vi "FPGAvi.vi"() -> ()   [LabVIEW 2014]
uses:
  <vilib>/Platform/TimedLoop/XDataNode/wakeup.ctl
  <vilib>/Platform/TimedLoop/XDataNode/XDNodeRunTimeDep.lvlib
  <vilib>/Platform/TimedLoop/XDataNode/nitl_modes.ctl
  <vilib>/Platform/TimedLoop/XDataNode/timing_clust.ctl
  <vilib>/Platform/TimedLoop/XDataNode/XDataNode.xnode
  <vilib>/eio/EIONode/EIONode.xnode
  <vilib>/rvi/eio/common/nirviEmuTemplateMethod_errors.vi
  <vilib>/rvi/DataTransferAndStorage/Container/XNode/niFpgaContainer.xnode
  <vilib>/rvi/FIFO/Fifo_Resource/nirvififoEmulationWrite.vi
  <vilib>/rvi/FIFO/Fifo_Resource/nirvififoEmulationRead.vi
  <vilib>/rvi/interface/RandomDataEmulation/nirviRandomDataFpgaReadWriteTemplate.vi
panel:
  out "DMA Overflow":bool
  in  "ADC A Requested":bool
  in  "ADC B Requested":bool
  in  "ADC C Requested":bool
  in  "ADC D Requested":bool
  in  "Acquire":bool
  out "Acquisition State":T1(ring)
  out "FIFO State":T2(ring)
  out "Init Done":bool
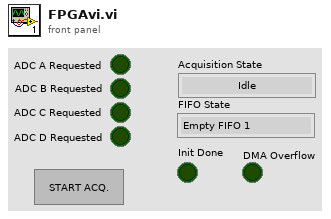
[diagram p1: front panel]
types:
  T1 = enum16{"Idle", "Determine Channel Selection", "Acquire", "Transfer"}
  T2 = enum16{"Empty FIFO 1", "Empty FIFO 2", "Empty FIFO 3", "Empty FIFO 4", "Empty FIFO 5", "Empty FIFO 6", "Empty FIFO 7", "Empty FIFO 8", "FIFO Read Complete"}
  T3 = typedef "XDNodeRunTimeDep.lvlib/timing_clust.ctl" = cluster{"Expected End [f-1]":u64, "Actual End [f-1]":u64, "Finished Late? [f-1]":bool, "Expected End [i-1]":u64, "Actual End [i-1]":u64, "Finished Late? [i-1]":bool, "Expected Start [i]":u64, "Actual Start [i]":u64, "Expected Start [f]":u64, "Actual Start [f]":u64, "Source Name":string, "Structure Name":string, "Period":i64, "Deadline":i64, "Offset":i64, "Start":i64, "Priority":i32, "Timeout":i32, "Mode":T4, "Wakeup Reason":T5, "Error":errorcluster, "Source Type":string, "Secondary Source Type":string, "Global End Time":u64, "Global Start Time":u64, "Frame Duration":u64, "Iteration Duration":u64, "Assigned CPU":i32, "I/O Scan Engine Mode":u32}
  T4 = typedef "XDNodeRunTimeDep.lvlib/nitl_modes.ctl" = enum32{"No Change", "Process missed periods, maintain original phase", "Discard missed periods, maintain original phase", "Process missed periods, ignore original phase", "Discard missed periods, ignore original phase"}
  T5 = typedef "XDNodeRunTimeDep.lvlib/wakeup.ctl" = enum32{"Normal", "Aborted", "Asynchronous wakeup", "Timing source error", "Timed loop error", "Timeout"}
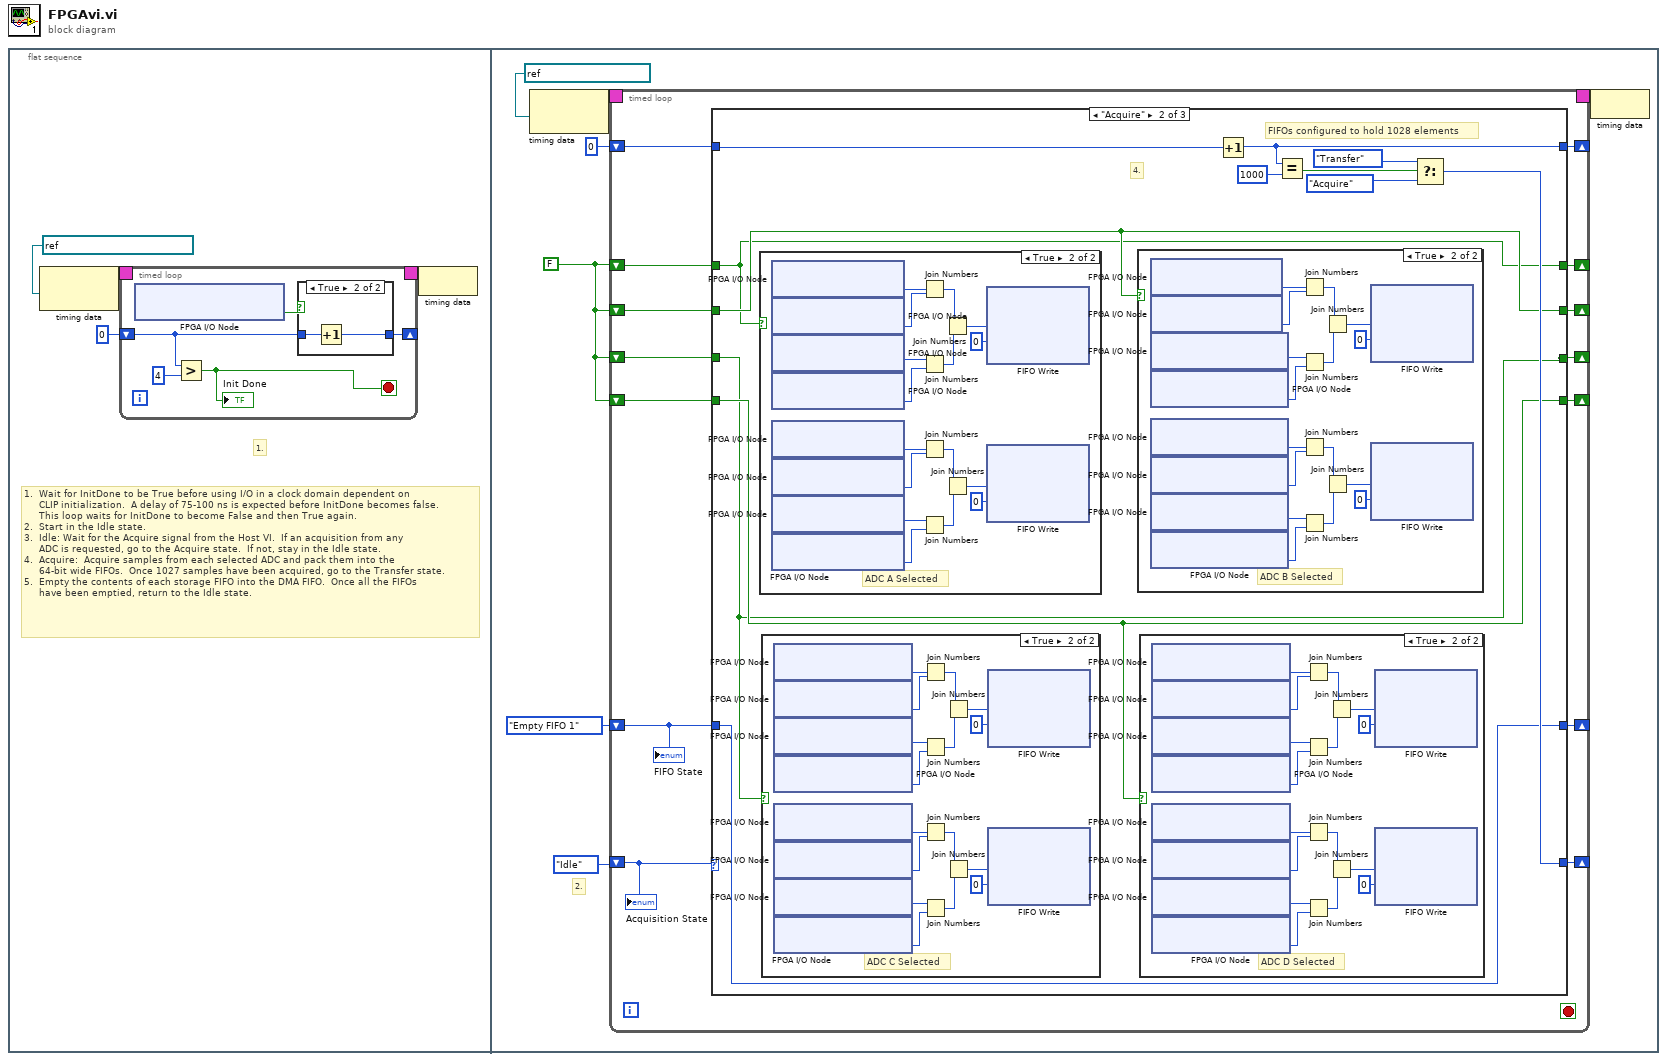
[diagram p0: block diagram]
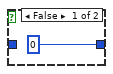
[diagram p2: hidden frame]
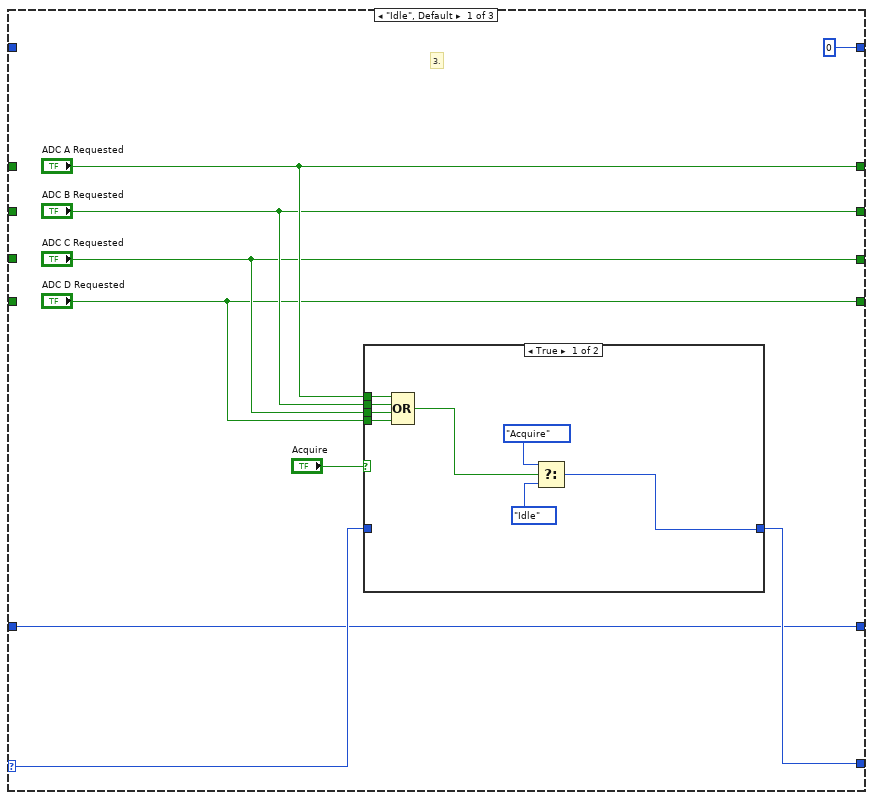
[diagram p3: hidden frame]
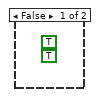
[diagram p5: hidden frame]
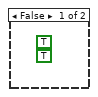
[diagram p6: hidden frame]
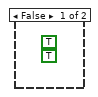
[diagram p7: hidden frame]
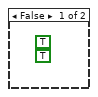
[diagram p8: hidden frame]
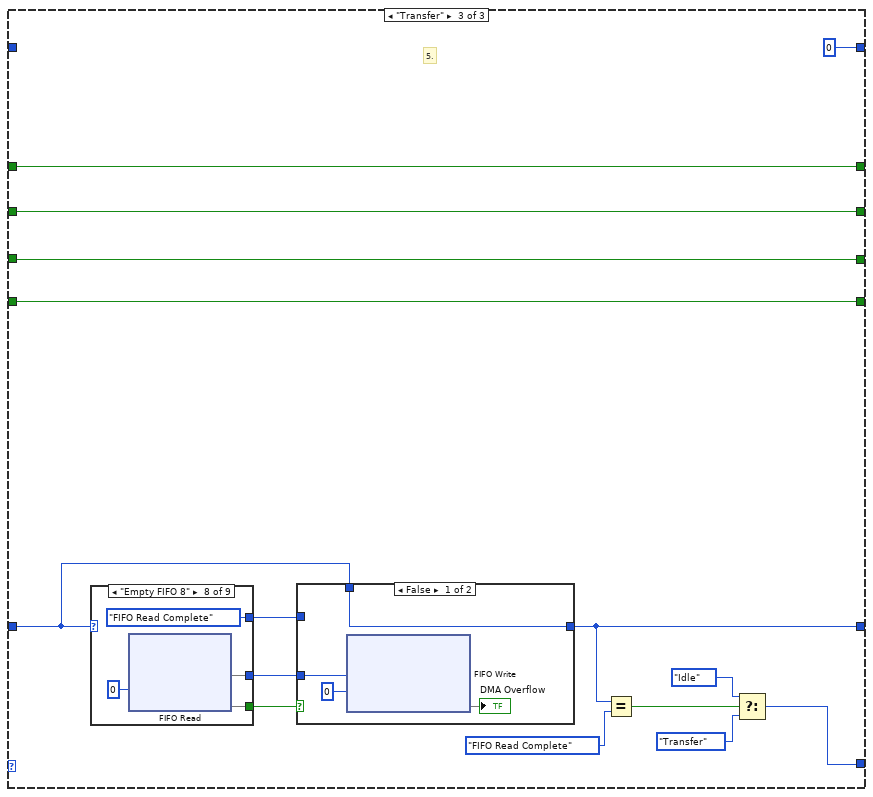
[diagram p9: hidden frame]
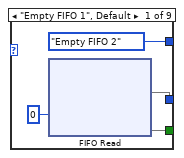
[diagram p11: hidden frame]
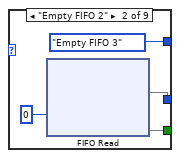
[diagram p12: hidden frame]
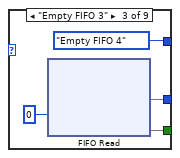
[diagram p13: hidden frame]
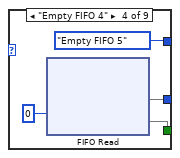
[diagram p14: hidden frame]
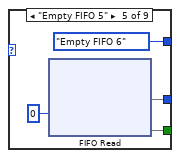
[diagram p15: hidden frame]
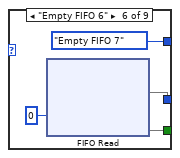
[diagram p16: hidden frame]
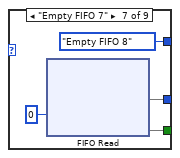
[diagram p17: hidden frame]
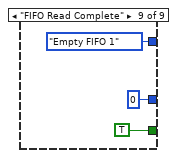
[diagram p18: hidden frame]
diagram:
  n1 = flat-sequence {
    frame #0 {
      # "1.  Wait for InitDone to be True before using I/O in a clock domain dependent on \n     CLIP initialization.  A delay of 75-100 ns is expected before InitDone becomes false.  \n     This loop waits for InitDone to become False and then True again.\n2.  Start in the Idle state. \n3.  Idle: Wait for the Acquire signal from the Host VI.  If an acquisition from any \n     ADC is requested, go to the Acquire state.  If not, stay in the Idle state.\n4.  Acquire:  Acquire samples from each selected ADC and pack them into the  \n     64-bit wide FIFOs.  Once 1027 samples have been acquired, go to the Transfer state.\n5.  Empty the contents of each storage FIFO into the DMA FIFO.  Once all the FIFOs \n     have been emptied, return to the Idle state."
      # "1."
      n2 = node-c288(refnum<k21> "40 MHz Onboard Clock" ("Source Name")) -> (w4:T3)
      n3 = timed-loop {
        shift-right: [w8] -> _
        shift-left: u16 0 -> [w7]
        timing: w4 -> [_]
        timing-out: [_] -> w3
        stop <- w5 stop-if-true
        n4 = xnode "FPGA I/O Node"() -> ("IO Module\\InitDone"=w9:bool)  [unwired: 1 in, 1 out]
        n5 = Greater?(x=w7, y=u16 4) -> (0:w5:bool)
        "Init Done" <- w5
        n6 = case shown="True" w9 {
          tunnel: [u16 0 w12] -> w8
          tunnel: w7 -> [_ w11]
          frame False {
          }
          frame True {
            n7 = Increment(x=w11) -> (x+1=w12:u16)
          }
        }
      }
      n8 = node-c288(w3) -> ()
    }
    frame #1 {
      w22 = FALSE
      # "2."
      n9 = node-c288(refnum<k21> "IO Module Clock 0" ("Source Name")) -> (w25:T3)
      n10 = timed-loop {
        timing: w25 -> [_]
        timing-out: [_] -> w24
        shift-right: [w31] -> _
        shift-left: T1."Idle" ("Acquisition State 2") -> [w28]
        shift-right: [w39] -> _
        shift-left: w22 -> [w35]
        shift-right: [w38] -> _
        shift-left: w22 -> [w34]
        shift-right: [w37] -> _
        shift-left: w22 -> [w33]
        shift-right: [w36] -> _
        shift-left: w22 -> [w32]
        shift-right: [w29] -> _
        shift-left: i16 0 -> [w30]
        shift-right: [w26] -> _
        shift-left: T2."Empty FIFO 1" -> [w27]
        stop <- _ stop-if-true
        n11 = case shown="\"Acquire\"" w28 {
          selector: w28 -> [w43 _ _]
          tunnel: [w48 w67 w137] -> w31
          tunnel: ["ADC A Requested" w59 w148] -> w39
          tunnel: ["ADC B Requested" w60 w147] -> w38
          tunnel: ["ADC C Requested" w61 w146] -> w37
          tunnel: ["ADC D Requested" w62 w145] -> w36
          tunnel: w35 -> [_ w59 w148]
          tunnel: w34 -> [_ w60 w147]
          tunnel: w33 -> [_ w61 w146]
          tunnel: w32 -> [_ w62 w145]
          tunnel: w30 -> [_ w66 _]
          tunnel: [i16 0 w63 i16 0] -> w29
          tunnel: w27 -> [w41 w58 w141]
          tunnel: [w41 w58 w138] -> w26
          frame "Idle", Default {
            # "3."
            n12 = case shown="True" "Acquire" {
              tunnel: "ADC D Requested" -> [w54 _]
              tunnel: "ADC C Requested" -> [w53 _]
              tunnel: "ADC B Requested" -> [w52 _]
              tunnel: "ADC A Requested" -> [w51 _]
              tunnel: [w50 w57] -> w48
              tunnel: w43 -> [_ w57]
              frame True {
                n13 = Compound Arithmetic op=OR(w51, w52, w53, w54) -> (w49:bool)
                n14 = Select(t=T1."Acquire" ("Acquisition State 2"), s=w49, f=T1."Idle" ("Acquisition State 2")) -> (s? t:f=w50:T1)
              }
              frame False {
              }
            }
          }
          frame "Acquire" {
            # "4."
            # "FIFOs configured to hold 1028 elements"
            n15 = case shown="True" w59 {
              frame False {
                (unwired) TRUE ("Timed Out?")
                (unwired) TRUE ("Timed Out?")
              }
              frame True {
                # "ADC A Selected"
                n16 = xnode "FPGA I/O Node"() -> ("IO Module\\AI A0"=w118:i16)  [unwired: 1 in, 1 out]
                n17 = xnode "FPGA I/O Node"() -> ("IO Module\\AI A1"=w119:i16)  [unwired: 1 in, 1 out]
                n18 = xnode "FPGA I/O Node"() -> ("IO Module\\AI A2"=w120:i16)  [unwired: 1 in, 1 out]
                n19 = xnode "FPGA I/O Node"() -> ("IO Module\\AI A3"=w121:i16)  [unwired: 1 in, 1 out]
                n20 = xnode "FPGA I/O Node"() -> ("IO Module\\AI A4"=w122:i16)  [unwired: 1 in, 1 out]
                n21 = xnode "FPGA I/O Node"() -> ("IO Module\\AI A5"=w123:i16)  [unwired: 1 in, 1 out]
                n22 = xnode "FPGA I/O Node"() -> ("IO Module\\AI A6"=w124:i16)  [unwired: 1 in, 1 out]
                n23 = xnode "FPGA I/O Node"() -> ("IO Module\\AI A7"=w125:i16)  [unwired: 1 in, 1 out]
                n24 = Join Numbers(hi=w118, lo=w119) -> ((hi.lo)=w129:u32)
                n25 = Join Numbers(hi=w120, lo=w121) -> ((hi.lo)=w128:u32)
                n26 = Join Numbers(hi=w122, lo=w123) -> ((hi.lo)=w132:u32)
                n27 = Join Numbers(hi=w124, lo=w125) -> ((hi.lo)=w133:u32)
                n28 = Join Numbers(hi=w129, lo=w128) -> ((hi.lo)=w127:u64)
                n29 = Join Numbers(hi=w132, lo=w133) -> ((hi.lo)=w131:u64)
                n30 = xnode ("FIFO Write")("Element"=w127, "Timeout"=0) -> ()  [unwired: 1 in, 2 out]
                n31 = xnode ("FIFO Write")("Element"=w131, "Timeout"=0) -> ()  [unwired: 1 in, 2 out]
              }
            }
            n32 = case shown="True" w61 {
              frame False {
                (unwired) TRUE ("Timed Out?")
                (unwired) TRUE ("Timed Out?")
              }
              frame True {
                # "ADC C Selected"
                n33 = xnode "FPGA I/O Node"() -> ("IO Module\\AI C16"=w86:i16)  [unwired: 1 in, 1 out]
                n34 = xnode "FPGA I/O Node"() -> ("IO Module\\AI C17"=w87:i16)  [unwired: 1 in, 1 out]
                n35 = xnode "FPGA I/O Node"() -> ("IO Module\\AI C18"=w88:i16)  [unwired: 1 in, 1 out]
                n36 = xnode "FPGA I/O Node"() -> ("IO Module\\AI C19"=w89:i16)  [unwired: 1 in, 1 out]
                n37 = xnode "FPGA I/O Node"() -> ("IO Module\\AI C20"=w90:i16)  [unwired: 1 in, 1 out]
                n38 = xnode "FPGA I/O Node"() -> ("IO Module\\AI C21"=w91:i16)  [unwired: 1 in, 1 out]
                n39 = xnode "FPGA I/O Node"() -> ("IO Module\\AI C22"=w92:i16)  [unwired: 1 in, 1 out]
                n40 = xnode "FPGA I/O Node"() -> ("IO Module\\AI C23"=w93:i16)  [unwired: 1 in, 1 out]
                n41 = Join Numbers(hi=w86, lo=w87) -> ((hi.lo)=w97:u32)
                n42 = Join Numbers(hi=w88, lo=w89) -> ((hi.lo)=w96:u32)
                n43 = Join Numbers(hi=w90, lo=w91) -> ((hi.lo)=w100:u32)
                n44 = Join Numbers(hi=w92, lo=w93) -> ((hi.lo)=w101:u32)
                n45 = Join Numbers(hi=w97, lo=w96) -> ((hi.lo)=w95:u64)
                n46 = Join Numbers(hi=w100, lo=w101) -> ((hi.lo)=w99:u64)
                n47 = xnode ("FIFO Write")("Element"=w95, "Timeout"=0) -> ()  [unwired: 1 in, 2 out]
                n48 = xnode ("FIFO Write")("Element"=w99, "Timeout"=0) -> ()  [unwired: 1 in, 2 out]
              }
            }
            n49 = case shown="True" w60 {
              frame False {
                (unwired) TRUE ("Timed Out?")
                (unwired) TRUE ("Timed Out?")
              }
              frame True {
                # "ADC B Selected"
                n50 = xnode "FPGA I/O Node"() -> ("IO Module\\AI B8"=w102:i16)  [unwired: 1 in, 1 out]
                n51 = xnode "FPGA I/O Node"() -> ("IO Module\\AI B9"=w103:i16)  [unwired: 1 in, 1 out]
                n52 = xnode "FPGA I/O Node"() -> ("IO Module\\AI B10"=w104:i16)  [unwired: 1 in, 1 out]
                n53 = xnode "FPGA I/O Node"() -> ("IO Module\\AI B11"=w105:i16)  [unwired: 1 in, 1 out]
                n54 = xnode "FPGA I/O Node"() -> ("IO Module\\AI B12"=w106:i16)  [unwired: 1 in, 1 out]
                n55 = xnode "FPGA I/O Node"() -> ("IO Module\\AI B13"=w107:i16)  [unwired: 1 in, 1 out]
                n56 = xnode "FPGA I/O Node"() -> ("IO Module\\AI B14"=w108:i16)  [unwired: 1 in, 1 out]
                n57 = xnode "FPGA I/O Node"() -> ("IO Module\\AI B15"=w109:i16)  [unwired: 1 in, 1 out]
                n58 = Join Numbers(hi=w102, lo=w103) -> ((hi.lo)=w113:u32)
                n59 = Join Numbers(hi=w104, lo=w105) -> ((hi.lo)=w112:u32)
                n60 = Join Numbers(hi=w106, lo=w107) -> ((hi.lo)=w116:u32)
                n61 = Join Numbers(hi=w108, lo=w109) -> ((hi.lo)=w117:u32)
                n62 = Join Numbers(hi=w113, lo=w112) -> ((hi.lo)=w111:u64)
                n63 = Join Numbers(hi=w116, lo=w117) -> ((hi.lo)=w115:u64)
                n64 = xnode ("FIFO Write")("Element"=w111, "Timeout"=0) -> ()  [unwired: 1 in, 2 out]
                n65 = xnode ("FIFO Write")("Element"=w115, "Timeout"=0) -> ()  [unwired: 1 in, 2 out]
              }
            }
            n66 = case shown="True" w62 {
              frame False {
                (unwired) TRUE ("Timed Out?")
                (unwired) TRUE ("Timed Out?")
              }
              frame True {
                # "ADC D Selected"
                n67 = xnode "FPGA I/O Node"() -> ("IO Module\\AI D24"=w70:i16)  [unwired: 1 in, 1 out]
                n68 = xnode "FPGA I/O Node"() -> ("IO Module\\AI D25"=w71:i16)  [unwired: 1 in, 1 out]
                n69 = xnode "FPGA I/O Node"() -> ("IO Module\\AI D26"=w72:i16)  [unwired: 1 in, 1 out]
                n70 = xnode "FPGA I/O Node"() -> ("IO Module\\AI D27"=w73:i16)  [unwired: 1 in, 1 out]
                n71 = xnode "FPGA I/O Node"() -> ("IO Module\\AI D28"=w74:i16)  [unwired: 1 in, 1 out]
                n72 = xnode "FPGA I/O Node"() -> ("IO Module\\AI D29"=w75:i16)  [unwired: 1 in, 1 out]
                n73 = xnode "FPGA I/O Node"() -> ("IO Module\\AI D30"=w76:i16)  [unwired: 1 in, 1 out]
                n74 = xnode "FPGA I/O Node"() -> ("IO Module\\AI D31"=w77:i16)  [unwired: 1 in, 1 out]
                n75 = Join Numbers(hi=w70, lo=w71) -> ((hi.lo)=w81:u32)
                n76 = Join Numbers(hi=w72, lo=w73) -> ((hi.lo)=w80:u32)
                n77 = Join Numbers(hi=w74, lo=w75) -> ((hi.lo)=w84:u32)
                n78 = Join Numbers(hi=w76, lo=w77) -> ((hi.lo)=w85:u32)
                n79 = Join Numbers(hi=w81, lo=w80) -> ((hi.lo)=w79:u64)
                n80 = Join Numbers(hi=w84, lo=w85) -> ((hi.lo)=w83:u64)
                n81 = xnode ("FIFO Write")("Element"=w79, "Timeout"=0) -> ()  [unwired: 1 in, 2 out]
                n82 = xnode ("FIFO Write")("Element"=w83, "Timeout"=0) -> ()  [unwired: 1 in, 2 out]
              }
            }
            n83 = Increment(x=w66) -> (x+1=w63:i16)
            n84 = Equal?(x=w63, y=i16 1000) -> (x = y?=w64:bool)
            n85 = Select(t=T1."Transfer" ("Acquisition State 2"), s=w64, f=T1."Acquire" ("Acquisition State 2")) -> (s? t:f=w67:T1)
          }
          frame "Transfer" {
            # "5."
            n86 = case shown="\"Empty FIFO 8\"" w141 {
              tunnel: [w156 w160 w163 w166 w171 w175 w180 w182 u64 0 ("Element")] -> w142
              tunnel: [w155 w159 w162 w167 w170 w174 w178 w183 TRUE ("Timed Out?")] -> w143
              tunnel: [T2."Empty FIFO 2" T2."Empty FIFO 3" T2."Empty FIFO 4" T2."Empty FIFO 5" T2."Empty FIFO 6" T2."Empty FIFO 7" T2."Empty FIFO 8" T2."FIFO Read Complete" T2."Empty FIFO 1"] -> w140
              frame "Empty FIFO 1", Default {
                n87 = xnode ("FIFO Read")("Timeout"=0) -> ("Element"=w156, "Timed Out?"=w155)  [unwired: 1 in, 1 out]
              }
              frame "Empty FIFO 2" {
                n88 = xnode ("FIFO Read")("Timeout"=0) -> ("Element"=w160, "Timed Out?"=w159)  [unwired: 1 in, 1 out]
              }
              frame "Empty FIFO 3" {
                n89 = xnode ("FIFO Read")("Timeout"=0) -> ("Element"=w163, "Timed Out?"=w162)  [unwired: 1 in, 1 out]
              }
              frame "Empty FIFO 4" {
                n90 = xnode ("FIFO Read")("Timeout"=0) -> ("Element"=w166, "Timed Out?"=w167)  [unwired: 1 in, 1 out]
              }
              frame "Empty FIFO 5" {
                n91 = xnode ("FIFO Read")("Timeout"=0) -> ("Element"=w171, "Timed Out?"=w170)  [unwired: 1 in, 1 out]
              }
              frame "Empty FIFO 6" {
                n92 = xnode ("FIFO Read")("Timeout"=0) -> ("Element"=w175, "Timed Out?"=w174)  [unwired: 1 in, 1 out]
              }
              frame "Empty FIFO 7" {
                n93 = xnode ("FIFO Read")("Timeout"=0) -> ("Element"=w180, "Timed Out?"=w178)  [unwired: 1 in, 1 out]
              }
              frame "Empty FIFO 8" {
                n94 = xnode ("FIFO Read")("Timeout"=0) -> ("Element"=w182, "Timed Out?"=w183)  [unwired: 1 in, 1 out]
              }
              frame "FIFO Read Complete" {
              }
            }
            n95 = case shown="False" w143 {
              tunnel: w142 -> [w152 _]
              tunnel: w140 -> [_ w153]
              tunnel: w141 -> [w151 _]
              tunnel: [w151 w153] -> w138
              frame False {
                n96 = xnode ("FIFO Write")("Element"=w152, "Timeout"=0) -> ("Timed Out?"=→"DMA Overflow")  [unwired: 1 in, 1 out]
              }
              frame True {
              }
            }
            n97 = Equal?(x=w138, y=T2."FIFO Read Complete") -> (x = y?=w134:bool)
            n98 = Select(t=T1."Idle" ("Acquisition State 2"), s=w134, f=T1."Transfer" ("Acquisition State 2")) -> (s? t:f=w137:T1)
          }
        }
        "Acquisition State" <- w28
        "FIFO State" <- w27
      }
      n99 = node-c288(w24) -> ()
    }
  }
